vi "Test.vi"() -> ()   [LabVIEW 2014]
uses:
  SensorData.ctl
  navXPacket.ctl
  EncoderPacket.ctl
  PotentiometerPacket.ctl
  distanceSensorPacket.ctl
  switchPacket.ctl
  SensorType.ctl
  SensorStatus.ctl
panel:
  out "Sensor Out":T1
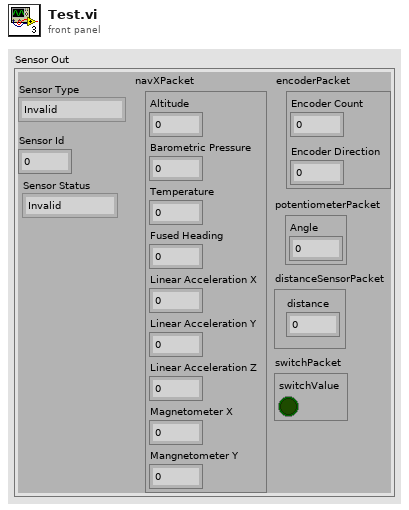
[diagram p1: front panel]
types:
  T1 = typedef "SensorData.ctl" = cluster{"Sensor Id":dbl, "navXPacket":T2, "encoderPacket":T3, "potentiometerPacket":T4, "distanceSensorPacket":T5, "switchPacket":T6, "Sensor Type":T7, "Sensor Status":T8}
  T2 = typedef "navXPacket.ctl" = cluster{"Altitude":dbl, "Barometric Pressure":dbl, "Fused Heading":dbl, "Linear Acceleration Y":dbl, "Linear Acceleration X":dbl, "Temperature":dbl, "Mangnetometer Y":dbl, "Magnetometer X":dbl, "Linear Acceleration Z":dbl}
  T3 = typedef "EncoderPacket.ctl" = cluster{"Encoder Count":dbl, "Encoder Direction":dbl}
  T4 = typedef "PotentiometerPacket.ctl" = cluster{"Angle":dbl}
  T5 = typedef "distanceSensorPacket.ctl" = cluster{"distance":dbl}
  T6 = typedef "switchPacket.ctl" = cluster{"switchValue":bool}
  T7 = typedef "SensorType.ctl" = enum16{"Invalid", "NavX", "Encoder", "Potentiometer", "Distance Sensor", "Switch"}
  T8 = typedef "SensorStatus.ctl" = enum16{"Invalid", "Operational", "Error occurred"}
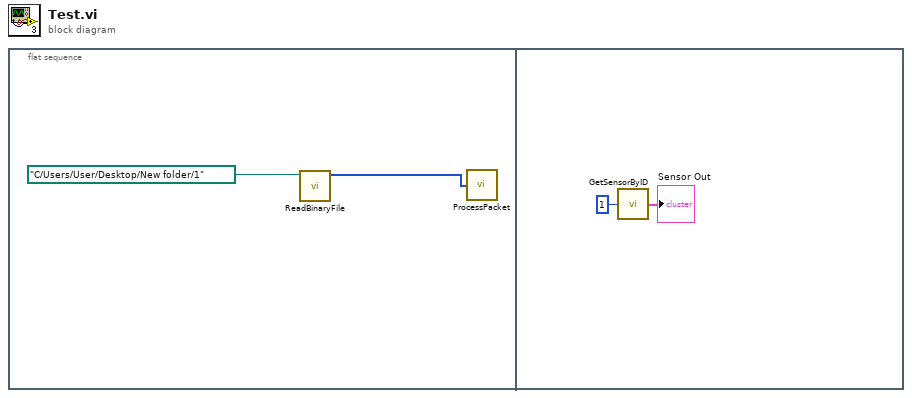
[diagram p0: block diagram]
diagram:
  n1 = flat-sequence {
    frame #0 {
      n2 = call "ReadBinaryFile.vi"("file path (use dialog)"=path "C:/Users/User/Desktop/New folder/1") -> ("byte array"=w2:u8[])  [unwired: 8 in, 1 out]
      n3 = call "ProcessPacket.vi"("Message"=w2) -> ()  [unwired: 5 in]
    }
    frame #1 {
      n4 = call "GetSensorByID.vi"("Sensor ID"=1) -> ("Sensor Out"=→"Sensor Out":T1)  [unwired: 4 in]
    }
  }
